vi "Ini key write (DBL).vi"(7 "Section":string, 8 "error in (no error)":errorcluster, 9 "Values (DBL)":dbl[](array[numeric]), 10 "Ini file interface":T2, 11 "Ini file refnum in":T1) -> (0 "error out":errorcluster, 3 "Ini file refnum out":T1)   [LabVIEW 2013]
uses:
  <vilib>/Utility/config.llb/Config Data RefNum.ctl
  Typedefs/Ini file interface (DBL).ctl
  <vilib>/Utility/config.llb/Write Key (Double).vi
  <vilib>/Utility/config.llb/Read Key (Double).vi
  <vilib>/Utility/config.llb/NI_LVConfig.lvlib
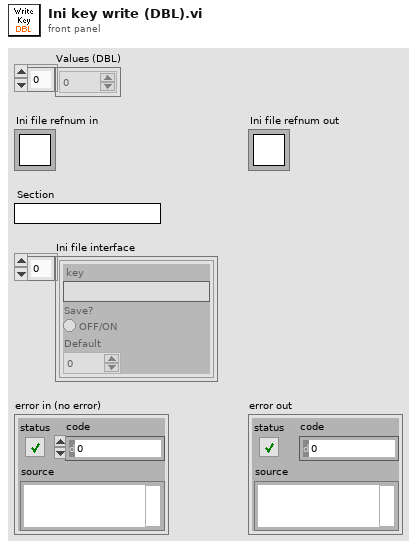
[diagram p1: front panel]
types:
  T1 = typedef "NI_LVConfig.lvlib/Config Data RefNum.ctl" = refnum<k1>
  T2 = typedef "Ini file interface (DBL).ctl" = cluster{"key":string, "Save?":bool, "Default":dbl}[]
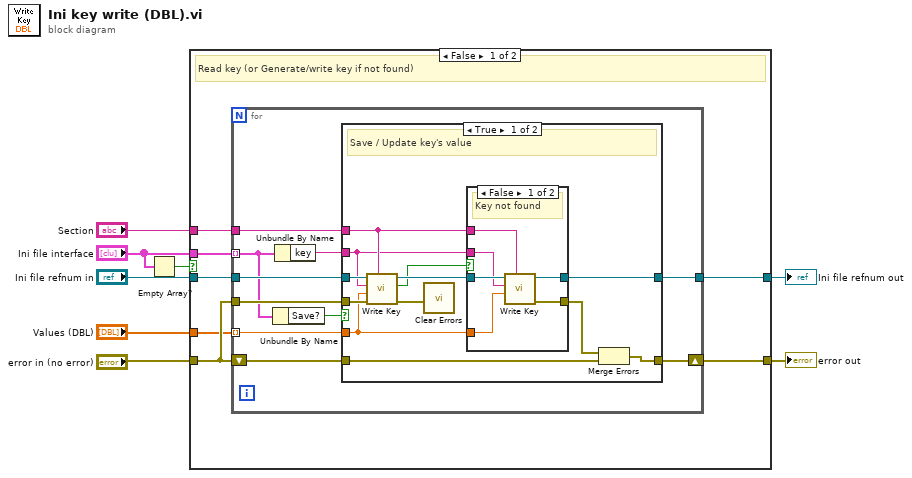
[diagram p0: block diagram]
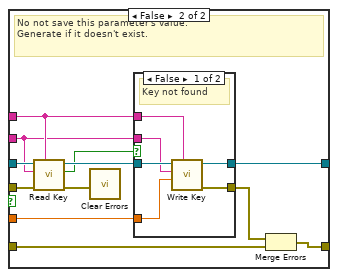
[diagram p3: hidden frame]
diagram:
  n1 = Empty Array?(array="Ini file interface") -> (empty?=w3:bool)
  n2 = case shown="False" w3 {
    tunnel: "Ini file refnum in" -> [w15 w65]
    tunnel: [w14 w65] -> w8
    tunnel: [w13 w64] -> w7
    tunnel: "error in (no error)" -> [w12 w64]
    tunnel: "Section" -> [w9 _]
    tunnel: "Ini file interface" -> [w11 _]
    tunnel: "Values (DBL)" -> [w10 _]
    frame False {
      # "Read key (or Generate/write key if not found)"
      n3 = for {
        tunnel: w15 -> [w25]
        tunnel: w12 -> [w24]
        tunnel: [w23] -> w14
        shift-right: [w22] -> w13
        shift-left: w12 -> [w21]
        tunnel: w11 -> [w17] mode=indexing
        tunnel: w10 -> [w20] mode=indexing
        tunnel: w9 -> [w19]
        n4 = Unbundle By Name(w17) -> ("Save?"=w16:bool)
        n5 = Unbundle By Name(w17) -> ("key"=w18:string)
        n6 = case shown="True" w16 {
          tunnel: w25 -> [w37 w56]
          tunnel: w24 -> [w36 w55]
          tunnel: [w27 w46] -> w23
          tunnel: [w35 w54] -> w22
          tunnel: w21 -> [w34 w53]
          tunnel: w18 -> [w30 w49]
          tunnel: w20 -> [w28 w47]
          tunnel: w19 -> [w31 w50]
          frame True {
            # "Save / Update key's value"
            n7 = call-poly <vilib>:"Write Key.vi"("section"=w31, "error in (no error)"=w36, "value"=w28, "key"=w30, "refnum"=w37) -> ("error out"=w33:errorcluster, "found?"=w26:bool, "refnum out"=w32:T1)  [unwired: 4 in]
            n8 = call <vilib>:"Clear Errors.vi"("error in (no error)"=w33) -> ()  [unwired: 6 in, 1 out]
            n9 = case shown="False" w26 {
              tunnel: w32 -> [w43 w44]
              tunnel: [w42 w44] -> w27
              tunnel: [w41 _] -> w29
              tunnel: w31 -> [w40 _]
              tunnel: w30 -> [w39 _]
              tunnel: w28 -> [w38 _]
              frame False {
                # "Key not found"
                n10 = call-poly <vilib>:"Write Key.vi"("section"=w40, "value"=w38, "key"=w39, "refnum"=w43) -> ("error out"=w41:errorcluster, "refnum out"=w42:T1)  [unwired: 5 in, 1 out]
              }
              frame True {
                # "Key found"
              }
            }
            n11 = Merge Errors(w29, w34) -> (w35:errorcluster)
          }
          frame False {
            # "No not save this parameter's value.\nGenerate if it doesn't exist."
            n12 = call-poly <vilib>:"Read Key.vi"("section"=w50, "error in (no error)"=w55, "key"=w49, "refnum"=w56) -> ("error out"=w52:errorcluster, "found?"=w45:bool, "refnum out"=w51:T1)  [unwired: 4 in, 1 out]
            n13 = call <vilib>:"Clear Errors.vi"("error in (no error)"=w52) -> ()  [unwired: 6 in, 1 out]
            n14 = case shown="False" w45 {
              tunnel: w51 -> [w62 w63]
              tunnel: [w61 w63] -> w46
              tunnel: [w60 _] -> w48
              tunnel: w50 -> [w59 _]
              tunnel: w49 -> [w58 _]
              tunnel: w47 -> [w57 _]
              frame False {
                # "Key not found"
                n15 = call-poly <vilib>:"Write Key.vi"("section"=w59, "value"=w57, "key"=w58, "refnum"=w62) -> ("error out"=w60:errorcluster, "refnum out"=w61:T1)  [unwired: 5 in, 1 out]
              }
              frame True {
                # "Key found"
              }
            }
            n16 = Merge Errors(w48, w53) -> (w54:errorcluster)
          }
        }
      }
    }
    frame True {
      # "Setup array is empty"
    }
  }
  "Ini file refnum out" <- w8
  "error out" <- w7
